vi "svc_Interpolate XY Data.vi"(6 "interpolated plot mapping":T1(ring), 7 "method":i32(ring)=1 items=["nearest", "linear", "spline", "cubic Hermite", "Lagrange"], 9 "test X":dbl[](array[numeric]), 10 "limit X":dbl[](array[numeric]), 11 "limit Y":dbl[](array[numeric])) -> (1 "xi used":dbl[](array[numeric]), 3 "yi":dbl[](array[numeric]))   [LabVIEW 2017]
uses:
  <vilib>/gmath/NI_Gmath.lvlib
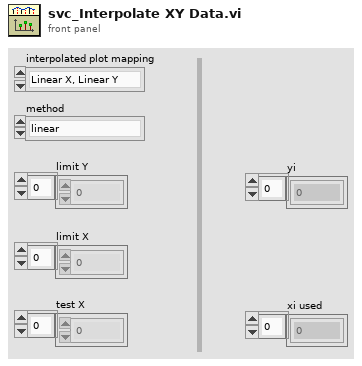
[diagram p1: front panel]
types:
  T1 = enum16{"Linear X, Linear Y", "Linear X, Log Y", "Log X, Linear Y", "Log X, Log Y"}
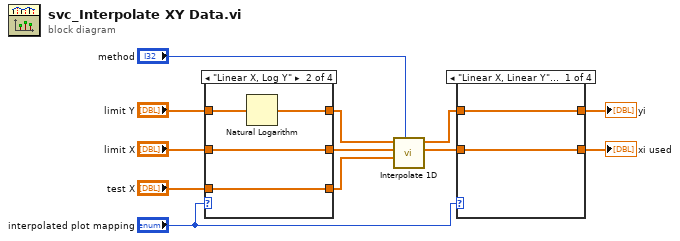
[diagram p0: block diagram]
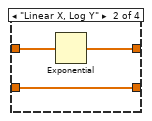
[diagram p2: hidden frame]
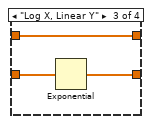
[diagram p3: hidden frame]
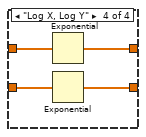
[diagram p4: hidden frame]
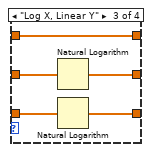
[diagram p6: hidden frame]
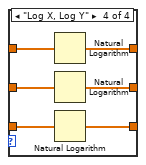
[diagram p7: hidden frame]
diagram:
  n1 = case shown="\"Linear X, Log Y\"" "interpolated plot mapping" {
    tunnel: "limit X" -> [w14 w19 w24 w30]
    tunnel: [w14 w19 w23 w27] -> w1
    tunnel: "test X" -> [w13 w18 w22 w29]
    tunnel: [w13 w18 w21 w28] -> w3
    tunnel: "limit Y" -> [w15 w17 w20 w26]
    tunnel: [w15 w16 w20 w25] -> w7
    frame "Linear X, Linear Y", Default {
    }
    frame "Linear X, Log Y" {
      n2 = Natural Logarithm(1:w17) -> (0:w16:dbl[])
    }
    frame "Log X, Linear Y" {
      n3 = Natural Logarithm(1:w24) -> (0:w23:dbl[])
      n4 = Natural Logarithm(1:w22) -> (0:w21:dbl[])
    }
    frame "Log X, Log Y" {
      n5 = Natural Logarithm(1:w26) -> (0:w25:dbl[])
      n6 = Natural Logarithm(1:w30) -> (0:w27:dbl[])
      n7 = Natural Logarithm(1:w29) -> (0:w28:dbl[])
    }
  }
  n8 = call <vilib>:"Interpolate 1D.vi"("method"="method", "xi"=w3, "X"=w1, "Y"=w7) -> ("xi used"=w6:dbl[], "yi"=w8:dbl[])  [unwired: 5 in, 1 out]
  n9 = case shown="\"Linear X, Linear Y\", Default" "interpolated plot mapping" {
    tunnel: w6 -> [w32 w35 w38 w42]
    tunnel: [w32 w35 w37 w41] -> w12
    tunnel: w8 -> [w31 w34 w36 w40]
    tunnel: [w31 w33 w36 w39] -> w9
    frame "Linear X, Linear Y", Default {
    }
    frame "Linear X, Log Y" {
      n10 = Exponential(1:w34) -> (0:w33:dbl[])
    }
    frame "Log X, Linear Y" {
      n11 = Exponential(1:w38) -> (0:w37:dbl[])
    }
    frame "Log X, Log Y" {
      n12 = Exponential(1:w40) -> (0:w39:dbl[])
      n13 = Exponential(1:w42) -> (0:w41:dbl[])
    }
  }
  "xi used" <- w12
  "yi" <- w9
